vi "Test Dynamic Method.vi"(8 "error in (no error)":errorcluster, 11 "Test Case Test Double Child with Override In":refnum<class "Test Case Test Double Child with Override.lvclass">) -> (0 "error out":errorcluster, 3 "Test Case Test Double Child with Override Out":refnum<class "Test Case Test Double Child with Override.lvclass">)   [LabVIEW 2020, in "Test Case Test Double Child with Override.lvclass"]
uses:
  Test Case Test Double Child with Override.lvclass
  C:/git/astemes-lunit/source/API/LUnit Test Case/LUnit Test Case.lvclass
  source/API/LUnit Test Case/LUnit Test Case.lvclass/LUnit Test Case.ctl
  source/API/LUnit Test Case/Private/Append Fail Result.vi
  source/API/LUnit Test Case/Private/Run In UI.vi
  <vilib>/Utility/error.llb/Clear Errors.vi
  source/API/LUnit Test Case/LUnit Test Case.lvclass
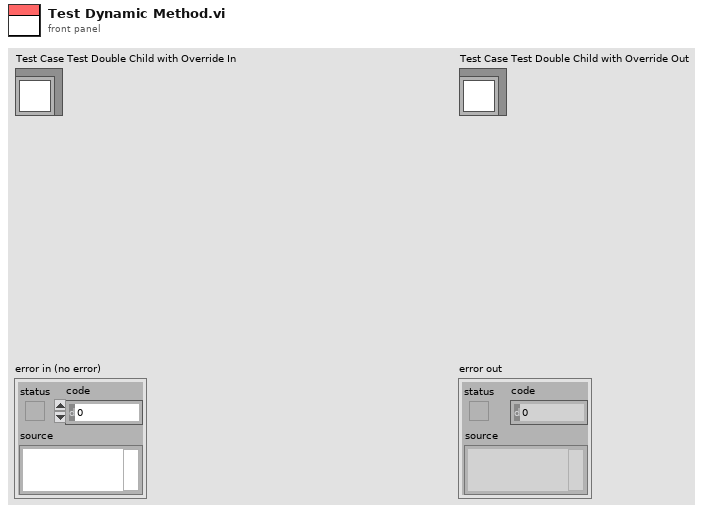
[diagram p1: front panel]
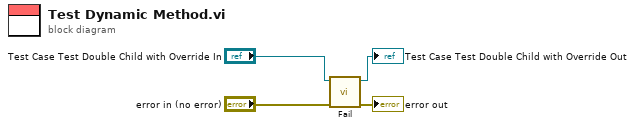
[diagram p0: block diagram]
diagram:
  n1 = call "Fail.vi"("error in (no error)"="error in (no error)", "LUnit Test Case In"="Test Case Test Double Child with Override In") -> ("error out"=→"error out":errorcluster, "LUnit Test Case Out"=→"Test Case Test Double Child with Override Out":refnum<class "Test Case Test Double Child with Override.lvclass">)  [unwired: 8 in]
